vi "_RT Update Lens Parameters.vi"(8 "error in":errorcluster, 10 "Lens":T1[](array[typedef])) -> (0 "error out":errorcluster)   [LabVIEW 2015]
uses:
  Type/_XML Lens.ctl
  Type/_RT Parameter.ctl
  Type/_RT Active Ch.ctl
  Type/_RT Expt.ctl
  Type/_Run Mode.ctl
  Type/_RT Mass Range.ctl
  Type/_RT Res Type.ctl
  _RT Global.vi
  <vilib>/Utility/error.llb/Error Cluster From Error Code.vi
  <vilib>/rvi/errors/niLvFpgaAdjustHostInterfaceError.vi
  <vilib>/rvi/interface/nirviReadWriteControl/nirviReadWriteControl.xnode
  Type/FPGA Typedef.ctl
  FPGA Bitfiles/FPGA9607.lvbitx
  NiFpgaLv.dll
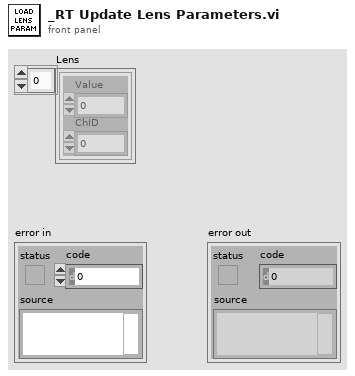
[diagram p1: front panel]
types:
  T1 = typedef "_XML Lens.ctl" = cluster{"Value":dbl, "ChID":u8}
  T2 = typedef "_RT Expt.ctl" = cluster{"StartT(mS)":i32, "#Cycles":i32, "Scan Type":T3, "PauseT(uS)":i32, "Polarity":u8, "DelayT(mS)":i32, "Active Ch":T4[], "Mass Range":T5[]}
  T3 = typedef "_Run Mode.ctl" = enum16{"MRM (Q1/Q2)", "Q1 Scan", "Q1 SRM", "Q2 Scan", "Q2 SRM", "Product Scan", "Precursor Scan", "Neutral Loss", "Neutral Gain"}
  T4 = typedef "_RT Active Ch.ctl" = cluster{"Start":i32, "Step":i32, "ChID":i32}
  T5 = typedef "_RT Mass Range.ctl" = cluster{"Steps":i32, "Dwell(uS)":i32, "Resolution Type":T6, "Ramping Ch":T4[]}
  T6 = typedef "_RT Res Type.ctl" = u16
  T7 = typedef "_RT Parameter.ctl" = cluster{"RunMode":i32, "Initial Ch":T4[], "Sync":u8, "Expt":T2[], "EqTime(mS)":i32}
  T8 = typedef "_RT Configuration 2.ctl" = cluster{"Name":string, "Ch#":u8, "Min":dbl, "Max":dbl, "Def+":dbl, "Def-":dbl, "Offset":dbl, "Slope":dbl, "Type":u8, "Description":string, "SettleT":dbl}
  T9 = typedef "FPGA Typedef.ctl" = refnum<k20>
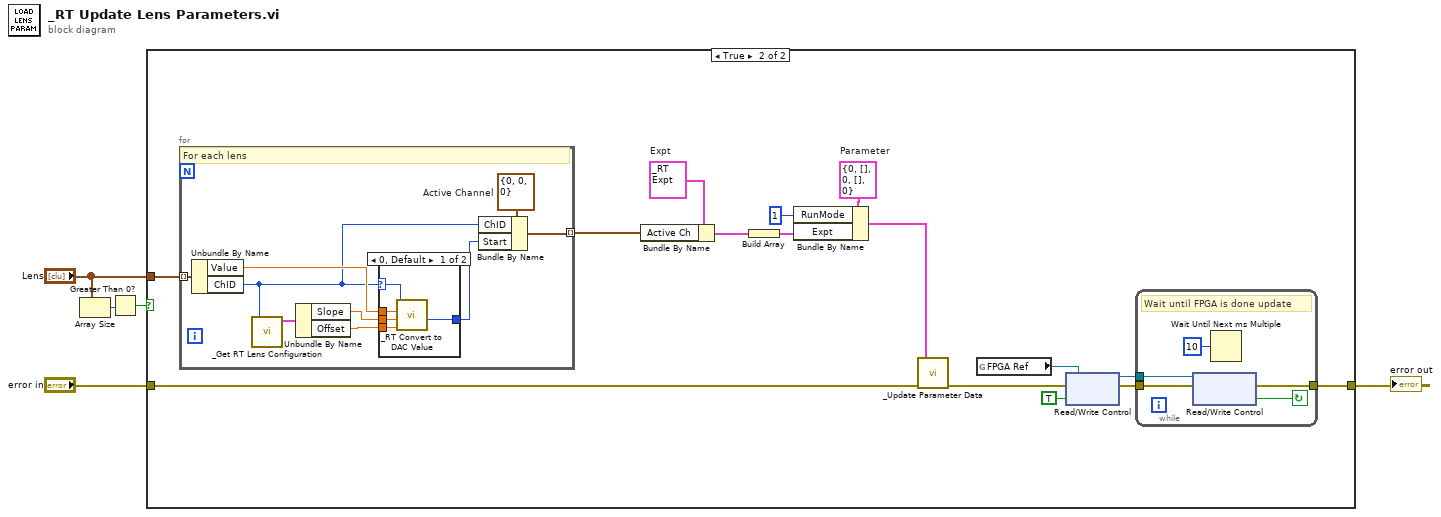
[diagram p0: block diagram]
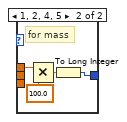
[diagram p3: hidden frame]
diagram:
  n1 = Array Size(array="Lens") -> (size(s)=w4:i32)
  n2 = Greater Than 0?(x=w4) -> (x > 0?=w3:bool)
  n3 = case shown="True" w3 {
    tunnel: "Lens" -> [_ w20]
    tunnel: "error in" -> [w6 w14]
    tunnel: [w6 w8] -> w1
    frame False {
    }
    frame True {
      w17 = T2 {"StartT(mS)"=0, "#Cycles"=1, "Scan Type"=enum."MRM (Q1/Q2)", "PauseT(uS)"=0, "Polarity"=0, "DelayT(mS)"=0, "Active Ch"=[], "Mass Range"=[]}  # Expt
      w19 = T7 {"RunMode"=0, "Initial Ch"=[], "Sync"=0, "Expt"=[], "EqTime(mS)"=0}  # Parameter
      n4 = for {
        tunnel: [w31] -> w21 mode=indexing
        tunnel: w20 -> [w30] mode=indexing
        w33 = T4 {"Start"=0, "Step"=0, "ChID"=0}  # Active Channel
        # "For each lens"
        n5 = Unbundle By Name(w30) -> ("Value"=w29:dbl, "ChID"=w28:u8)
        n6 = call "_Get RT Lens Configuration.vi"("Channel #"=w28) -> ("Lens Configuration"=w27:T8)  [unwired: 1 in, 5 out]
        n7 = Unbundle By Name(w27) -> ("Slope"=w35:dbl, "Offset"=w34:dbl)
        n8 = case shown="0, Default" w28 {
          selector: w28 -> [w36 _]
          tunnel: w29 -> [w40 w44]
          tunnel: w35 -> [w39 _]
          tunnel: w34 -> [w38 _]
          tunnel: [w37 w41] -> w32
          frame 0, Default {
            n9 = call "_RT Convert to DAC Value.vi"("Offset"=w38, "Slop"=w39, "Number"=w40, "Channel"=w36) -> ("DAC Value"=w37:i32)  [unwired: 7 in]
          }
          frame 1, 2, 4, 5 {
            # "for mass"
            n10 = Multiply(x=w44, y=100.0) -> (x*y=w42:dbl)
            n11 = To Long Integer(number=w42) -> (32bit integer=w41:i32)
          }
        }
        n12 = Bundle By Name(cluster=w33, "ChID"=w28, "Start"=w32) -> (w31:T4)
      }
      n13 = Bundle By Name(cluster=w17, "Active Ch"=w21) -> (w16:T2)
      n14 = Build Array(w16) -> (w15:T2[])
      n15 = Bundle By Name(cluster=w19, "RunMode"=1, "Expt"=w15) -> (w13:T7)
      n16 = call "_Update Parameter Data.vi"("error in"=w14, "Parameter"=w13) -> ("error out"=w12:errorcluster)  [unwired: 1 in, 4 out]
      n17 = global read "_RT Global.vi" "FPGA Ref"() -> (w11:T9)
      n18 = xnode "Read/Write Control"("FPGA VI Reference In"=w11, "error in"=w12, "Start"=TRUE) -> ("FPGA VI Reference Out"=w7:T9, "error out"=w9:errorcluster)
      n19 = while {
        tunnel: w9 -> [w26]
        tunnel: [w25] -> w8
        tunnel: w7 -> [w24]
        stop <- w23 continue-if-true
        # "Wait until FPGA is done update"
        n20 = xnode "Read/Write Control"("FPGA VI Reference In"=w24, "error in"=w26) -> ("error out"=w25:errorcluster, "Running"=w23:bool)  [unwired: 1 out]
        n21 = Wait Until Next ms Multiple(millisecond multiple=u32 10) -> ()  [unwired: 1 out]
      }
    }
  }
  "error out" <- w1
